vi "edge_thresh.vi"(10 "threshold":dbl=2.0, 11 "input cluster":cluster{sgl[], dbl[]}) -> (1 "miny":sgl, 2 "midy":sgl, 3 "maxy":sgl)   [LabVIEW 2018]
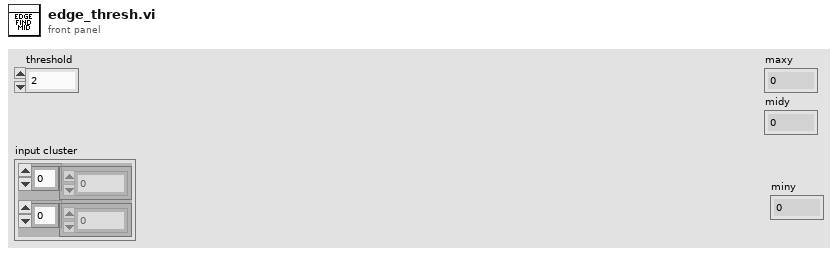
[diagram p1: front panel]
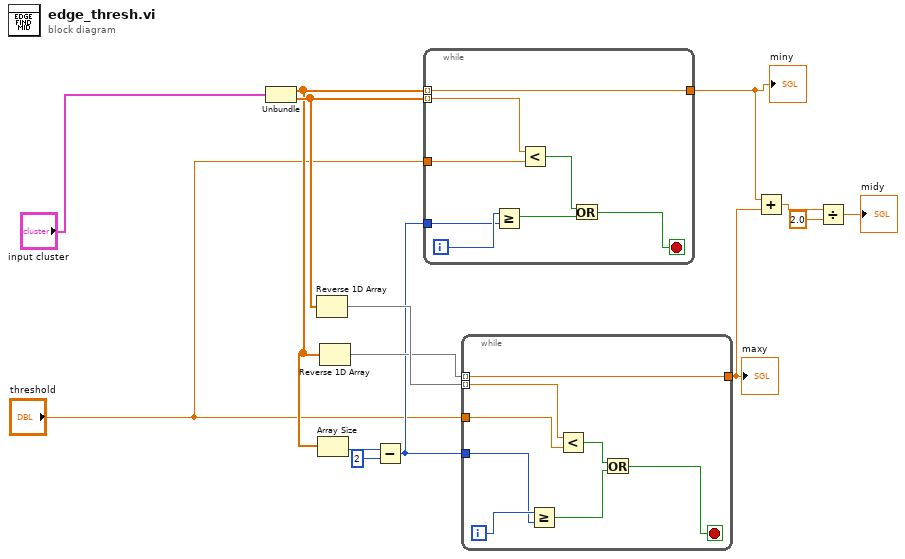
[diagram p0: block diagram]
diagram:
  n1 = Unbundle("input cluster") -> (w5:sgl[], w13:dbl[])
  n2 = Reverse 1D Array(array=w13) -> (reversed array=w12:dbl[])
  n3 = Array Size(array=w5) -> (size(s)=w4:i32)
  n4 = Reverse 1D Array(array=w5) -> (reversed array=w11:sgl[])
  n5 = Subtract(x=w4, y=2) -> (x-y=w2:i32)
  n6 = while {
    tunnel: w13 -> [w22] mode=indexing
    tunnel: w5 -> [w21] mode=indexing
    tunnel: [w21] -> w10
    tunnel: w2 -> [w19]
    tunnel: "threshold" -> [w15]
    i -> [w20]
    stop <- w16 stop-if-true
    n7 = Greater Or Equal?(x=w20, y=w19) -> (x >= y?=w18:bool)
    n8 = Less?(x=w22, y=w15) -> (x < y?=w17:bool)
    n9 = Or(x=w17, y=w18) -> (x .or. y?=w16:bool)
  }
  "miny" <- w10
  n10 = while {
    tunnel: w12 -> [w30] mode=indexing
    tunnel: w11 -> [w28] mode=indexing
    tunnel: [w28] -> w9
    tunnel: w2 -> [w27]
    tunnel: "threshold" -> [w23]
    i -> [w29]
    stop <- w24 stop-if-true
    n11 = Greater Or Equal?(x=w29, y=w27) -> (x >= y?=w25:bool)
    n12 = Less?(x=w30, y=w23) -> (x < y?=w26:bool)
    n13 = Or(x=w26, y=w25) -> (x .or. y?=w24:bool)
  }
  "maxy" <- w9
  n14 = Add(x=w10, y=w9) -> (x+y=w8:sgl)
  n15 = Divide(x=w8, y=sgl 2.0) -> (x/y=→"midy":sgl)
